vi "Update Sub Build Spec.vi"(0 "NI Build Specification in":refnum<class "NI Build Specification_LV.lvclass">, 5 "Sub Build Spec":refnum<class "NI Build Specification_LV.lvclass">, 11 "error in (no error)":errorcluster) -> (4 "NI Build Specification out":refnum<class "NI Build Specification_LV.lvclass">, 15 "error out":errorcluster)   [LabVIEW 2017, in "CL_G3_VIComponentBuilder.lvlib" / "NI Build Specification_LV.lvclass"]
doc: "Updates a build spec in the <Anchor><Text>Sub Build Specs</Text><AnchorName>Sub Build Specs</AnchorName><PageName>NI Build Specification_LV Class Documentation</PageName><Space>TCS</Space></Anchor> lookup table."
uses:
  NI Build Specification_LV.lvclass
  NI Build Specification_LV.lvclass/NI Build Specification_LV.ctl
  Accessors/Read Export's Build Spec Name.vi
  Accessors/Read Sub Build Specs.vi
  Accessors/Write Sub Build Specs.vi
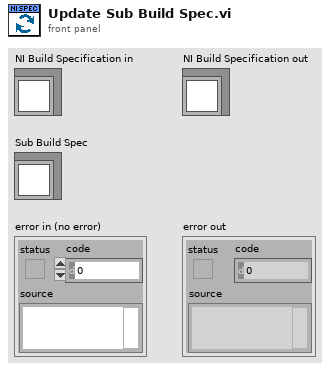
[diagram p1: front panel]
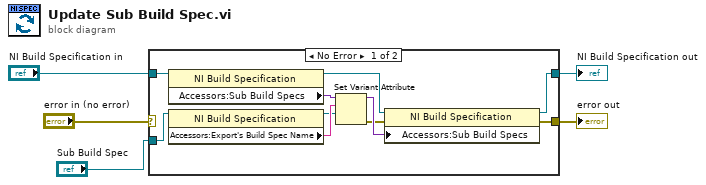
[diagram p0: block diagram]
diagram:
  n1 = case shown="No Error" "error in (no error)" {
    selector: "error in (no error)" -> [_ w17]
    tunnel: [w6 w17] -> w4
    tunnel: [w13 w16] -> w2
    tunnel: "NI Build Specification in" -> [w15 w16]
    tunnel: "Sub Build Spec" -> [w10 _]
    frame No Error {
      n2 = property class="NI Build Specification"(reference=w15) -> (reference out=w14:refnum<class "NI Build Specification_LV.lvclass">, "Accessors:Sub Build Specs"=w12:variant)  [unwired: 1 in, 1 out]
      n3 = property class="NI Build Specification"(reference=w10) -> (reference out=w8:refnum<class "NI Build Specification_LV.lvclass">, "Accessors:Export's Build Spec Name"=w9:string)  [unwired: 1 in, 1 out]
      n4 = Set Variant Attribute(Variant=w12, name=w9, value=w8) -> (Variant out=w11:variant, error out=w7:errorcluster)  [unwired: 1 in, 1 out]
      n5 = property class="NI Build Specification"(reference=w14, error in=w7, "Accessors:Sub Build Specs"=w11) -> (reference out=w13:refnum<class "NI Build Specification_LV.lvclass">, error out=w6:errorcluster)
    }
    frame Error {
    }
  }
  "error out" <- w4
  "NI Build Specification out" <- w2
